vi "Boolean Counter.vi"(1 "Reset":bool, 2 "Initial Count":i64, 3 "Count Down":bool, 4 "Count Up":bool) -> (0 "Count":i64)   [LabVIEW 2012]
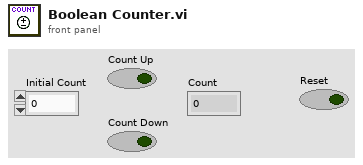
[diagram p1: front panel]
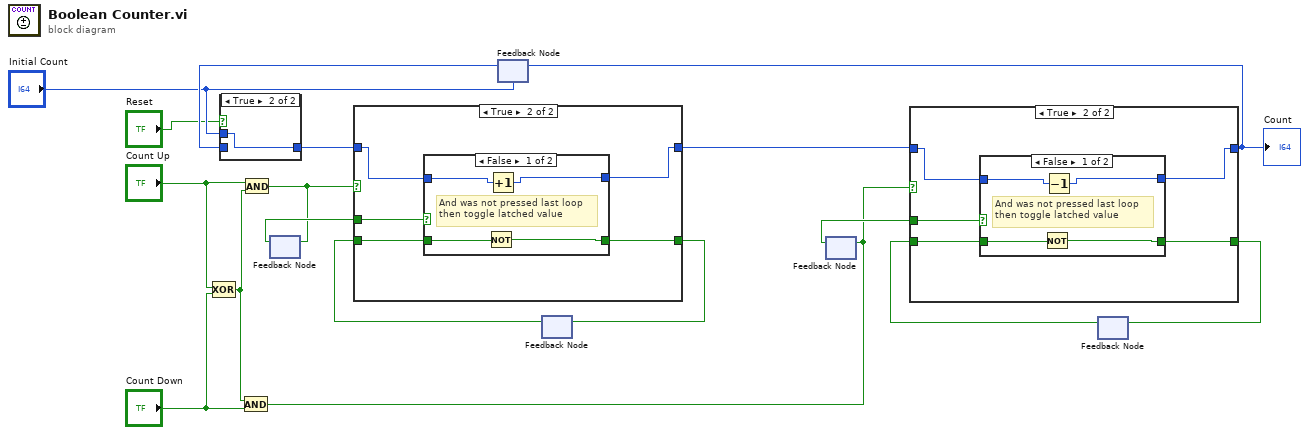
[diagram p0: block diagram]
diagram:
  n1 = Compound Arithmetic op=XOR("Count Up", "Count Down") -> (w6:bool)
  n2 = And(x=w6, y="Count Down") -> (x .and. y?=w7:bool)
  n3 = And(x="Count Up", y=w6) -> (x .and. y?=w9:bool)
  n4 = feedback #1() -> (w17:bool)  [unwired: 1 out]
  n5 = feedback-in #1(w9) -> ()
  n6 = feedback #2("Initial Count") -> (w4:i64)
  n7 = case shown="True" "Reset" {
    tunnel: w4 -> [w18 _]
    tunnel: [w18 w19] -> w3
    tunnel: "Initial Count" -> [_ w19]
    frame False {
    }
    frame True {
    }
  }
  n8 = feedback #3() -> (w15:bool)  [unwired: 1 out]
  n9 = case shown="True" w9 {
    tunnel: [w21 w26] -> w16
    tunnel: w17 -> [_ w24]
    tunnel: w15 -> [w21 w25]
    tunnel: w3 -> [w20 w23]
    tunnel: [w20 w22] -> w11
    frame False {
      # "then do nothing"
      # "If button is not pressed"
    }
    frame True {
      n10 = case shown="False" w24 {
        tunnel: [w30 w32] -> w26
        tunnel: w25 -> [w29 w32]
        tunnel: w23 -> [w27 w31]
        tunnel: [w28 w31] -> w22
        frame False {
          # "And was not pressed last loop\nthen toggle latched value"
          n11 = Not(x=w29) -> (.not. x?=w30:bool)
          n12 = Increment(x=w27) -> (x+1=w28:i64)
        }
        frame True {
          # "And was pressed last loop\nthen hold current latched value"
        }
      }
    }
  }
  n13 = feedback-in #3(w16) -> ()
  n14 = feedback #4() -> (w12:bool)  [unwired: 1 out]
  n15 = feedback-in #4(w7) -> ()
  n16 = feedback #5() -> (w14:bool)  [unwired: 1 out]
  n17 = case shown="True" w7 {
    tunnel: [w34 w39] -> w13
    tunnel: w12 -> [_ w37]
    tunnel: w14 -> [w34 w38]
    tunnel: w11 -> [w33 w36]
    tunnel: [w33 w35] -> w10
    frame False {
      # "then do nothing"
      # "If button is not pressed"
    }
    frame True {
      n18 = case shown="False" w37 {
        tunnel: [w43 w45] -> w39
        tunnel: w38 -> [w42 w45]
        tunnel: w36 -> [w40 w44]
        tunnel: [w41 w44] -> w35
        frame False {
          # "And was not pressed last loop\nthen toggle latched value"
          n19 = Not(x=w42) -> (.not. x?=w43:bool)
          n20 = Decrement(x=w40) -> (x-1=w41:i64)
        }
        frame True {
          # "And was pressed last loop\nthen hold current latched value"
        }
      }
    }
  }
  "Count" <- w10
  n21 = feedback-in #2(w10) -> ()
  n22 = feedback-in #5(w13) -> ()
